vi "SortOnKey (SubVI).vi"(6 "error out":errorcluster, 7 "Unsorted Array":dbl[][](array[numeric]), 8 "Descending?":bool=TRUE, 9 "Sort by column...":u32=2) -> (4 "error out 2":errorcluster, 5 "Sorted array":dbl[][](array[numeric]))   [LabVIEW 2011]
doc: "This vi sorts a 2D array according to the elements in an specified column. JacobKers09"
panel:
  out "Sort column values":dbl[](graph)
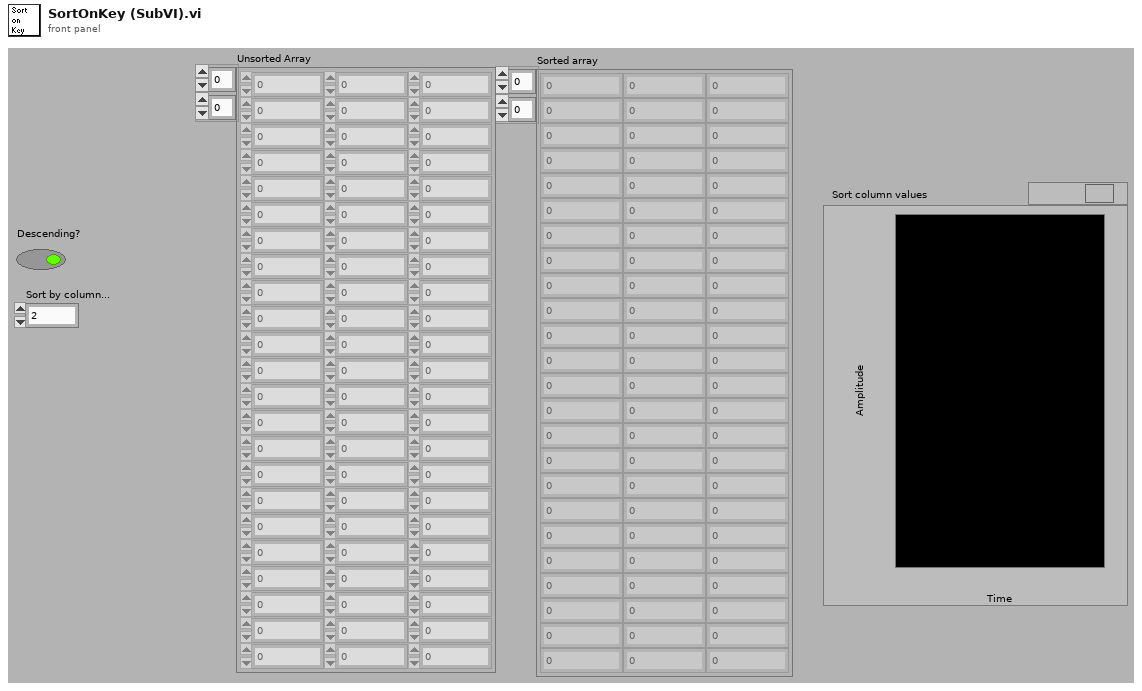
[diagram p1: front panel]
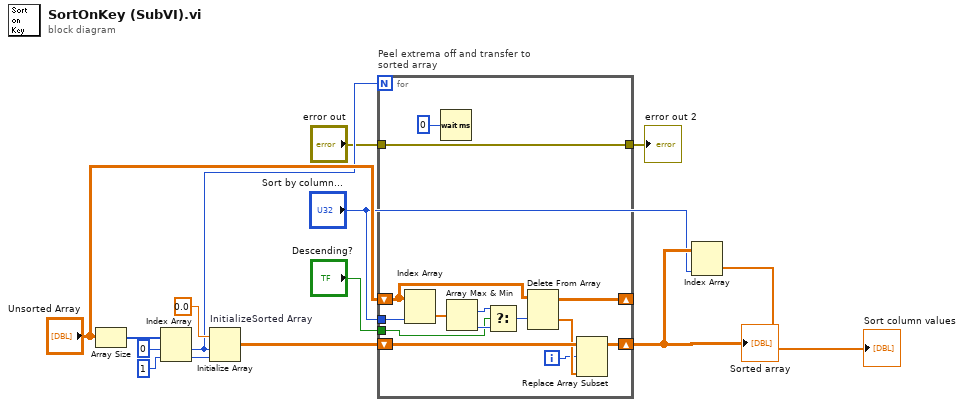
[diagram p0: block diagram]
diagram:
  n1 = Array Size(array="Unsorted Array") -> (size(s)=w12:i32[])
  n2 = Index Array(array=w12, index #1=0 ("index"), index #2=1 ("index")) -> (element #1=w7:i32, element #2=w8:i32)
  n3 = Initialize Array "InitializeSorted Array"(0.0 ("element"), w7, w8) -> (w6:dbl[][])
  n4 = for "Peel extrema off and transfer to \nsorted array" {
    N: w7 -> [_]
    tunnel: "Descending?" -> [w26]
    shift-right: [w24] -> _
    shift-left: "Unsorted Array" -> [w17]
    shift-right: [w20] -> w3
    shift-left: w6 -> [w23]
    tunnel: "error out" -> [w19]
    tunnel: [w19] -> w4
    tunnel: "Sort by column..." -> [w16]
    i -> [w21]
    n5 = Index Array(array=w17, index (col)=w16) -> (element=w15:dbl[])  [unwired: 1 in]
    n6 = Wait (ms)(milliseconds to wait=u32 0) -> ()  [unwired: 1 out]
    n7 = Array Max & Min(array=w15) -> (max index (indices)=w28:i32, min index (indices)=w27:i32)  [unwired: 2 out]
    n8 = Select(t=w28, s=w26, f=w27) -> (s? t:f=w25:i32)
    n9 = Delete From Array(array=w17, index (row)=w25) -> (deleted portion=w22:dbl[], array with subset deleted=w24:dbl[][])  [unwired: 2 in]
    n10 = Replace Array Subset(array=w23, new element=w22, index (row)=w21) -> (w20:dbl[][])  [unwired: 1 in]
  }
  "Sorted array" <- w3
  "error out 2" <- w4
  n11 = Index Array(array=w3, index (col)="Sort by column...") -> (element=→"Sort column values":dbl[])  [unwired: 1 in]
